vi "Release Session.vi"(8 "error in":errorcluster, 10 "force destroy? (F)":bool, 11 "File DVR":T1) -> (0 "error out":errorcluster, 2 "Session Destroyed?":bool)   [LabVIEW 2014, in "File Session.lvclass"]
doc: "Release the session associated with the current reference. If this is the last reference in the session or if the user specifies to force a destroy, we will close the file associated with the reference. If the reference is no good, then we will not close it."
uses:
  File Session.lvclass
  <userlib>/_Session Fwk/Session - Root.lvclass
  File Session DVR.ctl
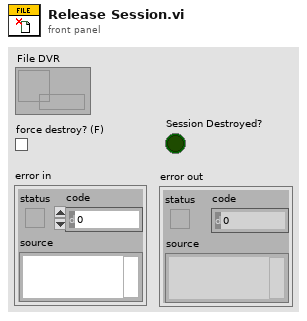
[diagram p1: front panel]
types:
  T1 = typedef "File Session.lvclass/File Session DVR.ctl" = refnum<data-value>
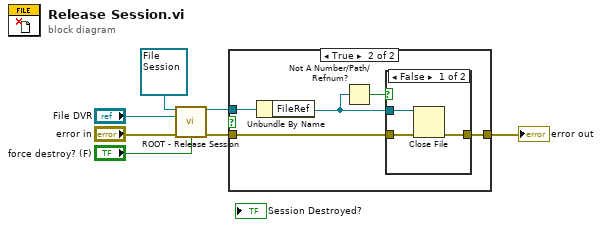
[diagram p0: block diagram]
diagram:
  n1 = call <userlib>:"ROOT - Release Session.vi"("OBJ - Session in"=refnum<class "File Session.lvclass"> refnum ("File Session in"), "Session Handle in"="File DVR", "error in (no error)"="error in", "force destroy? (F)"="force destroy? (F)") -> ("OBJ - Session out"=w4:refnum<class "File Session.lvclass">, "error out"=w2:errorcluster)  [unwired: 10 in]
  n2 = case shown="True" {
    selector: _ -> [_ _]
    tunnel: w4 -> [_ w13]
    tunnel: w2 -> [w8 w12]
    tunnel: [w8 w11] -> w1
    frame False {
    }
    frame True {
      n3 = Unbundle By Name(w13) -> ("FileRef"=w10:refnum<file>)
      n4 = Not A Number/Path/Refnum?(number/path/refnum=w10) -> (NaN/Path/Refnum?=w9:bool)
      n5 = case shown="False" w9 {
        tunnel: w12 -> [w16 w17]
        tunnel: [w15 w17] -> w11
        tunnel: w10 -> [w14 _]
        frame False {
          n6 = Close File(refnum=w14, error in=w16) -> (error out=w15:errorcluster)  [unwired: 1 out]
        }
        frame True {
        }
      }
    }
  }
  "error out" <- w1
